vi "Set Letter Time.vi"(8 "error in (no error)":errorcluster, 9 "Time":dbl[unit], 10 "Letter":string, 11 "CS++PPG in":refnum<class "CS++PPG.lvclass">) -> (0 "error out":errorcluster, 3 "CS++PPG out":refnum<class "CS++PPG.lvclass">)   [LabVIEW 2015, in "CS++PPG.lvlib" / "CS++PPG.lvclass"]
doc: "This VI sets a new time value for a given letter of the timing pattern. This should also work while the pulsed pattern generator is running."
uses:
  CS++PPG.lvclass
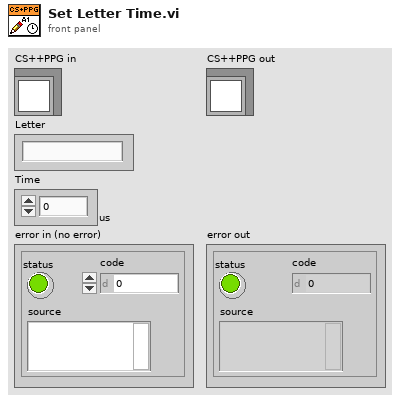
[diagram p1: front panel]
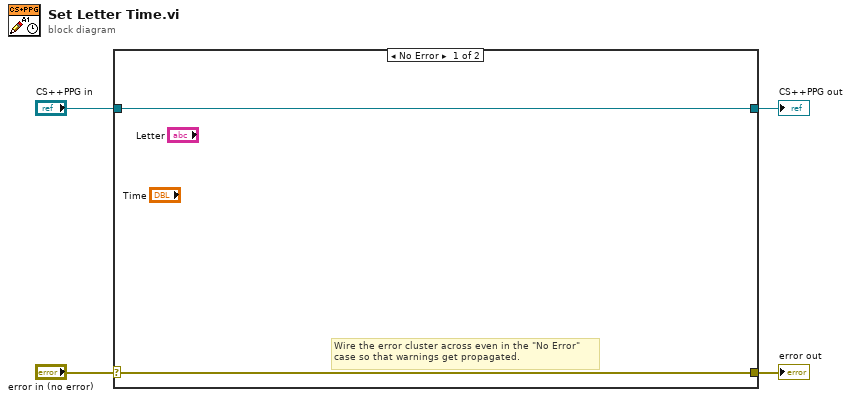
[diagram p0: block diagram]
diagram:
  n1 = case shown="No Error" "error in (no error)" {
    selector: "error in (no error)" -> [w5 w8]
    tunnel: [w5 w8] -> w3
    tunnel: [w6 w7] -> w1
    tunnel: "CS++PPG in" -> [w6 w7]
    frame No Error {
      # "Wire the error cluster across even in the \"No Error\"\ncase so that warnings get propagated."
    }
    frame Error {
    }
  }
  "error out" <- w3
  "CS++PPG out" <- w1
